vi "Average7Revised.vi"() -> ()   [LabVIEW 2016]
panel:
  in  "7":dbl format="%#_13g"
  in  "6":dbl format="%#_13g"
  in  "5":dbl format="%#_13g"
  out "average!!":dbl
  in  "4":dbl
  in  "3":dbl
  in  "2":dbl
  in  "1":dbl
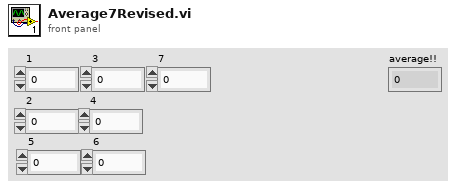
[diagram p1: front panel]
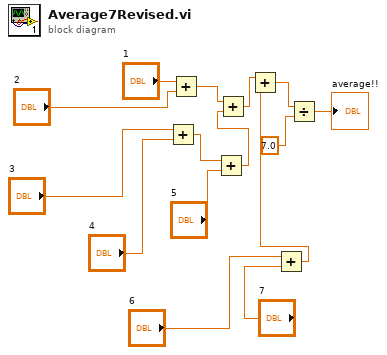
[diagram p0: block diagram]
diagram:
  n1 = Add(x="3", y="4") -> (x+y=w8:dbl)
  n2 = Add(x="1", y="2") -> (x+y=w15:dbl)
  n3 = Add(x=w8, y="5") -> (x+y=w7:dbl)
  n4 = Add(x=w15, y=w7) -> (x+y=w5:dbl)
  n5 = Add(x="6", y="7") -> (x+y=w3:dbl)
  n6 = Add(x=w5, y=w3) -> (x+y=w4:dbl)
  n7 = Divide(x=w4, y=7.0) -> (x/y=→"average!!":dbl)
